vi "2019-05-09_whileLoop.vi"() -> ()   [LabVIEW 2018]
panel:
  out "Loop Counter":i32
  in  "Stop Button":bool
  out "Match?":bool
  in  "숫자형 컨트롤":dbl
  out "Current Number":dbl
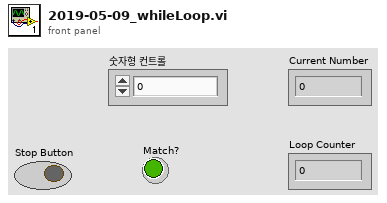
[diagram p1: front panel]
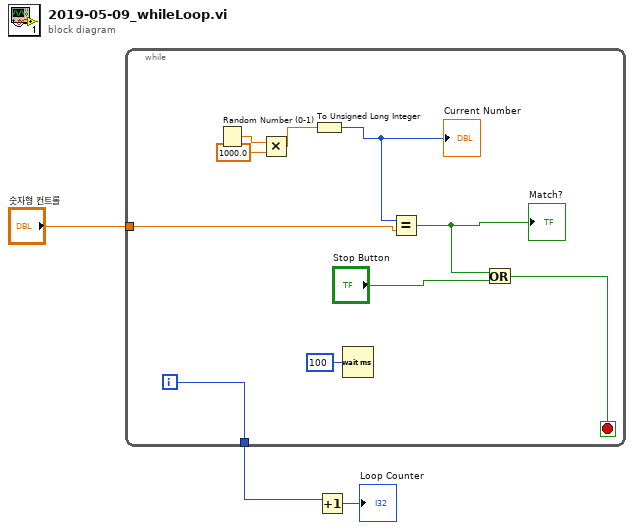
[diagram p0: block diagram]
diagram:
  n1 = while {
    tunnel: "숫자형 컨트롤" -> [w9]
    tunnel: [w5] -> w2
    i -> [w5]
    stop <- w6 stop-if-true
    n2 = Random Number (0-1)() -> (number: 0 to 1=w13:dbl)
    n3 = Multiply(x=w13, y=1000.0) -> (x*y=w11:dbl)
    n4 = To Unsigned Long Integer(number=w11) -> (unsigned 32bit integer=w10:u32)
    "Current Number" <- w10
    n5 = Wait (ms)(milliseconds to wait=u32 100 ("대기 시간 (ms)")) -> ()  [unwired: 1 out]
    n6 = Equal?(x=w10, y=w9) -> (x = y?=w8:bool)
    "Match?" <- w8
    n7 = Or(x=w8, y="Stop Button") -> (x .or. y?=w6:bool)
  }
  n8 = Increment(x=w2) -> (x+1=→"Loop Counter":i32)
